vi "Get cif_manager_LauncherStatus.vi"(8 "error in (no error)":errorcluster, 11 "gRPCid":T1) -> (0 "error out":errorcluster, 2 "package_templatemessage":T2, 3 "gRPCid out":T1)   [LabVIEW 2021, in "CIF_Launcher_server.lvlib"]
uses:
  CIF_Launcher_server.lvlib
  cif_manager_LauncherStatus.ctl
  cif_manager_LauncherInfo.ctl
  cif_manager_LauncherType.ctl
  cif_common_Status.ctl
  <vilib>/gRPC/LabVIEW gRPC Library/Shared/grpcId.ctl
  cif_manager_LauncherStatus_Flat.ctl
  cif_manager_LauncherInfo_Flat.ctl
  cif_common_Status_Flat.ctl
  2ed25e12-861d-4677-8ead-ace2906b2041.vi
  <vilib>/gRPC/LabVIEW gRPC Library/Shared/TranslateGrpcError.vi
  FlatToRichcif_manager_LauncherInfo.vi
  FlatToRichcif_common_Status.vi
  <vilib>/gRPC/LabVIEW gRPC Library/Server API/Server/Get Server DLL Path.vi
  <vilib>/Utility/error.llb/Error Cluster From Error Code.vi
  <vilib>/gRPC/LabVIEW gRPC Library/grpc-lvsupport-release.lvlib
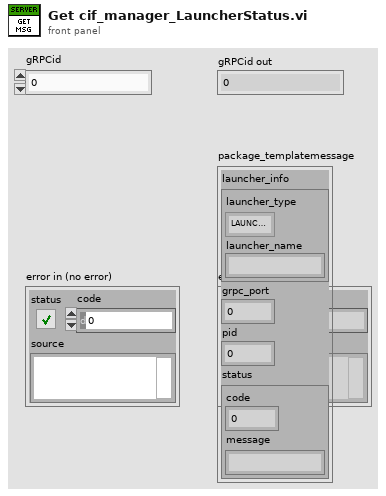
[diagram p1: front panel]
types:
  T1 = typedef "grpc-lvsupport-release.lvlib/grpcId.ctl" = u64
  T2 = typedef "CIF_Launcher_server.lvlib/cif_manager_LauncherStatus.ctl" = cluster{"launcher_info":T3, "grpc_port":i32, "pid":u32, "status":T5}
  T3 = typedef "CIF_Launcher_server.lvlib/cif_manager_LauncherInfo.ctl" = cluster{"launcher_type":T4, "launcher_name":string}
  T4 = typedef "CIF_Launcher_server.lvlib/cif_manager_LauncherType.ctl" = enum32{"LAUNCHERTYPE_UNKNOWN", "LAUNCHERTYPE_LABVIEW"}
  T5 = typedef "CIF_Launcher_server.lvlib/cif_common_Status.ctl" = cluster{"code":i32, "message":string}
  T6 = typedef "CIF_Launcher_server.lvlib/cif_manager_LauncherStatus_Flat.ctl" = cluster{"launcher_info":T7, "grpc_port":i32, "pid":u32, "status":T8}
  T7 = typedef "CIF_Launcher_server.lvlib/cif_manager_LauncherInfo_Flat.ctl" = cluster{"launcher_type":T4, "launcher_name":string}
  T8 = typedef "CIF_Launcher_server.lvlib/cif_common_Status_Flat.ctl" = cluster{"code":i32, "message":string}
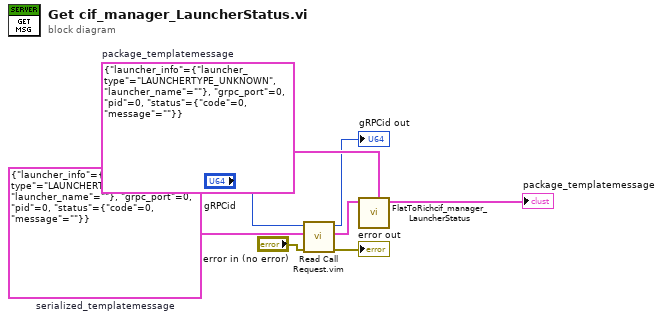
[diagram p0: block diagram]
diagram:
  w6 = T6 {"launcher_info"={"launcher_type"=enum."LAUNCHERTYPE_UNKNOWN", "launcher_name"=""}, "grpc_port"=0, "pid"=0, "status"={"code"=0, "message"=""}}  # serialized_templatemessage
  w5 = T2 {"launcher_info"={"launcher_type"=enum."LAUNCHERTYPE_UNKNOWN", "launcher_name"=""}, "grpc_port"=0, "pid"=0, "status"={"code"=0, "message"=""}}  # package_templatemessage
  n1 = call "Read Call Request.vim"("error in"="error in (no error)", "Request Type"=w6, "gRPCid in"="gRPCid") -> ("error out"=→"error out":errorcluster, "Request Data"=w4:T6, "gRPCid out"=→"gRPCid out":T1)  [unwired: 6 in]
  n2 = call "FlatToRichcif_manager_LauncherStatus.vi"("OutputClusterType"=w5, "InputCluster"=w4) -> ("OutputCluster"=→"package_templatemessage":T2)  [unwired: 9 in]
